vi "Manipulation3_1.vi"() -> ()   [LabVIEW 2017]
panel:
  out "Boolean 3":bool
  out "Boolean 2":bool
  out "Boolean":bool
  in  "stop":bool
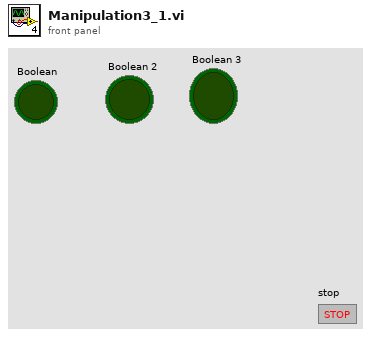
[diagram p1: front panel]
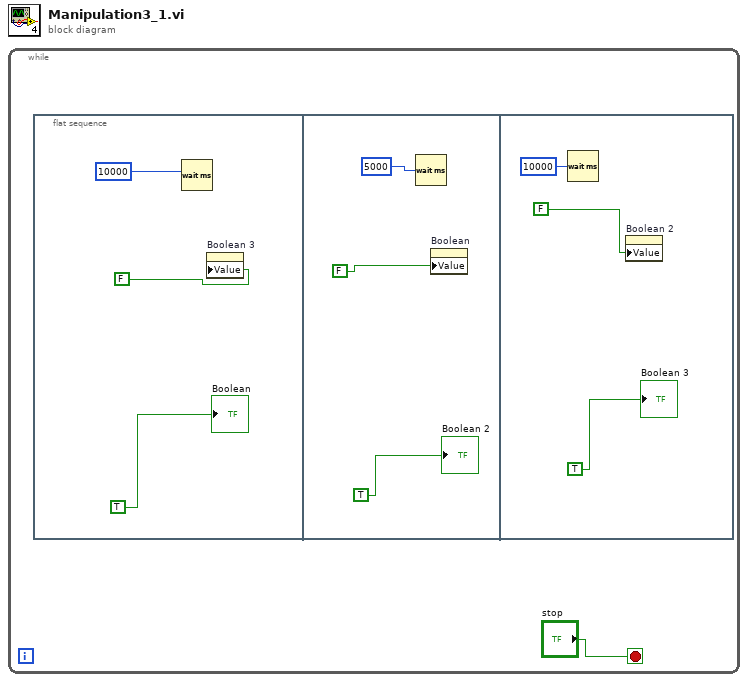
[diagram p0: block diagram]
diagram:
  n1 = while {
    stop <- "stop" stop-if-true
    n2 = flat-sequence {
      frame #0 {
        n3 = Wait (ms)(milliseconds to wait=10000) -> ()  [unwired: 1 out]
        n4 = property on="Boolean 3" class="Bool (strict)"("Value"=FALSE) -> ()  [unwired: 2 in, 2 out]
        "Boolean" <- TRUE
      }
      frame #1 {
        n5 = Wait (ms)(milliseconds to wait=5000) -> ()  [unwired: 1 out]
        n6 = property on="Boolean" class="Bool (strict)"("Value"=FALSE) -> ()  [unwired: 2 in, 2 out]
        "Boolean 2" <- TRUE
      }
      frame #2 {
        n7 = Wait (ms)(milliseconds to wait=10000) -> ()  [unwired: 1 out]
        n8 = property on="Boolean 2" class="Bool (strict)"("Value"=FALSE) -> ()  [unwired: 2 in, 2 out]
        "Boolean 3" <- TRUE
      }
    }
  }
